vi "pam.vi"() -> ()   [LabVIEW 2016]
panel:
  out "Waveform Graph 3":dynamicdata(graph)
  out "Waveform Graph 2":dynamicdata(graph)
  out "Waveform Graph":dynamicdata(graph)
  in  "Frequency 2":dbl(knob)=10.1 caption="Frequency" scale=0.0..500.0
  in  "Frequency":dbl(knob)=10.1 scale=0.0..100.0
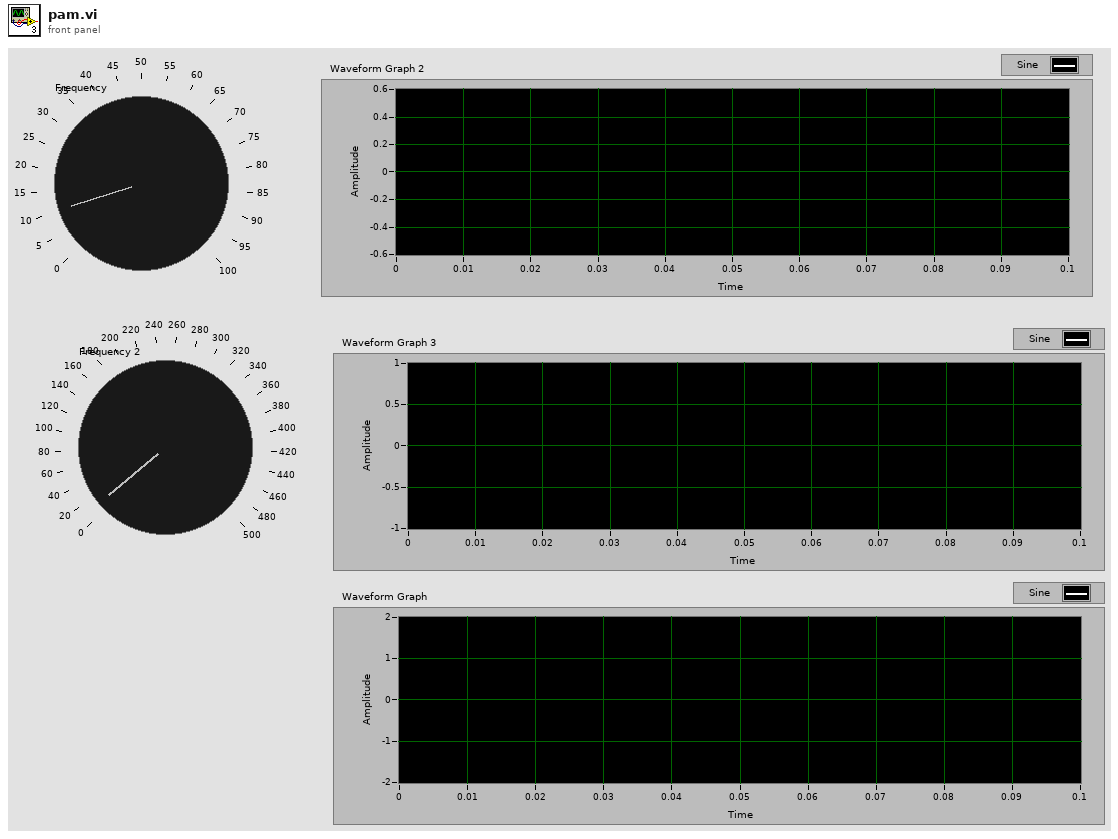
[diagram p1: front panel]
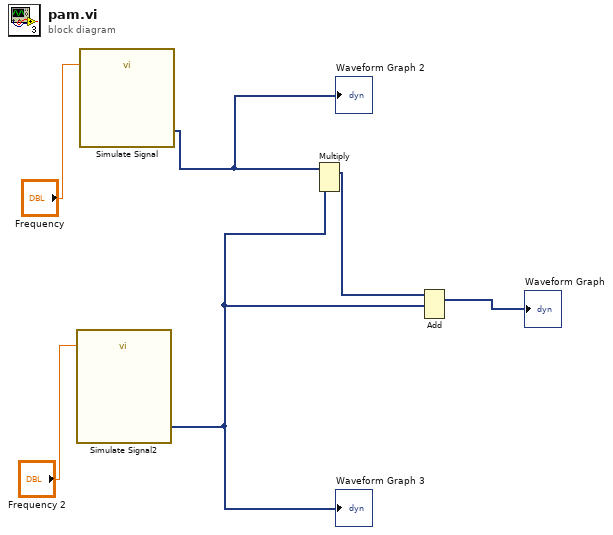
[diagram p0: block diagram]
diagram:
  n1 = call "Simulate Signal2"("Frequency"="Frequency 2") -> ("Sine"=w2:dynamicdata)  [unwired: 13 in, 1 out]
  "Waveform Graph 3" <- w2
  n2 = call "Simulate Signal"("Frequency"="Frequency") -> ("Sine"=w1:dynamicdata)  [unwired: 13 in, 1 out]
  "Waveform Graph 2" <- w1
  n3 = Multiply(1:w2, 2:w1) -> (0:w4:dynamicdata)  [unwired: 1 in, 1 out]
  n4 = Add(1:w2, 2:w4) -> (0:→"Waveform Graph":dynamicdata)  [unwired: 1 in, 1 out]
